vi "PushPull.vi"(6 "speed_uL_s":dbl, 7 "pushTo":string, 9 "volume_uL":dbl, 10 "pullFrom":string, 11 ".NET Refnum in":refnum<k24>) -> (3 ".NET Refnum out":refnum<k24>)   [LabVIEW 2020]
uses:
  C:/Users/bashc/Desktop/ChannelAutomatorR_.05/PumpAdapter.exe
  PumpAdapter.exe
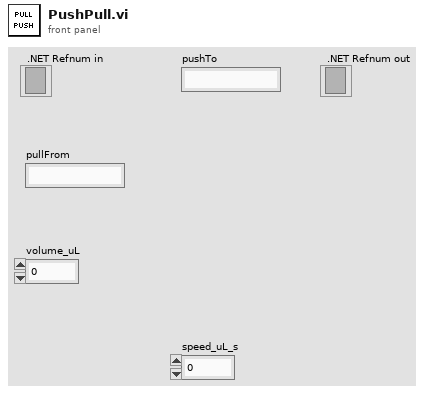
[diagram p1: front panel]
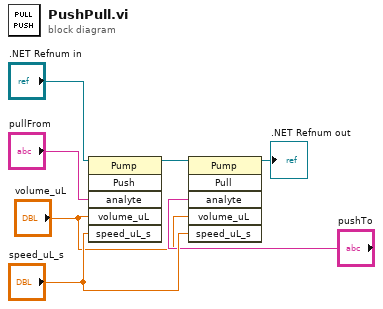
[diagram p0: block diagram]
diagram:
  n1 = invoke class="Pump" method="Push"(reference=".NET Refnum in", "analyte"="pullFrom", "volume_uL"="volume_uL", "speed_uL_s"="speed_uL_s") -> (reference out=w2:refnum<k24>)  [unwired: 2 in, 5 out]
  n2 = invoke class="Pump" method="Pull"(reference=w2, "analyte"="pushTo", "volume_uL"="volume_uL", "speed_uL_s"="speed_uL_s") -> (reference out=→".NET Refnum out":refnum<k24>)  [unwired: 2 in, 5 out]
